vi "Selection ActionBuilder.vi"(9 "Selection Action":T4, 10 "Isolate HPBD":bool, 11 "Chamber Selection":T3) -> (2 "Command Array Out":T1[](array[typedef]), 3 "Action Array Out":T2[](array[typedef]))   [LabVIEW 2011]
uses:
  Selection Action_typdef.ctl
  Chamber Selection_typdef.ctl
  action_typdef.ctl
  command_typdef.ctl
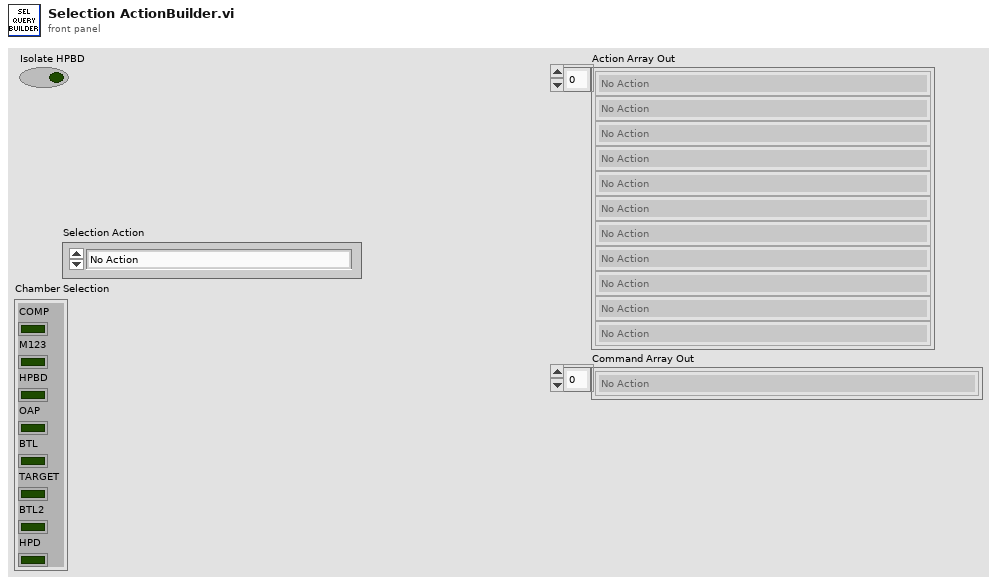
[diagram p1: front panel]
types:
  T1 = typedef "command_typdef.ctl" = enum16{"No Action", "Set GPM Mode LB", "EXIT GPM Mode LB", "Set GPM Mode EC", "EXIT GPM Mode EC", "Set GVM mode LB", "Set GVM Mode EC", "Open LB Backing Valve", "Open EC Backing Valve", "Open EC Roughing Valve", "Open LB Roughing Valve", "Open M123 Roughing Valve", "Close M123 Roughing Valve", "Open Compressor Roughing Valve", "Close Compressor Roughing Valve", "Open BeamDump Roughing Valve", "Close BeamDump Roughing Valve", "Open OAP Roughing Valve", "Close OAP Roughing Valve", "Open BTL Roughing Valve", "Close BTL Roughing Valve", "Open Target Roughing Valve", "Close Target Roughing Valve", "Open BTL2 Roughing Valve", "Close BTL2 Roughing Valve", "Open HPD Roughing Valve", "Close HPD Roughing Valve", "LB Start Roughing Pump ", "EC Start Roughing Pump", "Open COMP Turbo Backing Valve", "Open M123 Turbo Backing Valve", "Open OAP Turbo Backing Valve", "Open HPBD Turbo Backing Valve", "Open BLT Turbo Backing Valve", "Open TARGET1 Turbo Backing Valve", "Open TARGET2 Turbo Backing Valve", "Open BLT2 Turbo Backing Valve", "Open HPD Turbo Backing Valve", "LB Start Turbo Backing Pump", "EC Start Turbo Backing Pump", "Start COMP Turbo Pump", "Start M123 Turbo Pump", "Start OAP Turbo Pump", "Start BTL Turbo Pump", "Start TARGET1 Turbo Pump", "Start TARGET2 Turbo Pump", "Start BTL2 Turbo Pump", "Start HPD Turbo Pump", "Open COMP Turbo Gate Valve", "Open M123 Turbo Gate Valve", "Open OAP Turbo Gate Valve", "Open BTL Turbo Gate Valve", "Open TARGET1 Turbo Gate Valve", "Open TARGET2 Turbo Gate Valve", "Open BTL2 Turbo Gate Valve", "Open HPD Turbo Gate Valve"}
  T2 = typedef "action_typdef.ctl" = enum16{"No Action", "Is EC GPM Mode ON?", "Is EC GPM Mode Off?", "Is EC GVM Mode ON?", "Is EC GVM Off?", "Is  EC GPM or GVM Mode ON?", "Is LB GPM Mode ON?", "Is LB GPM Mode Off?", "Is LB GVM Mode ON?", "Is LB GVM Mode Off?", "Is  LB GPM or GVM Mode ON?", "Is M123 Turbo Gate Valve Opened? ", "Is M123 Turbo Gate Valve Closed?", "Is OAP Turbo Gate Valve Opened?", "Is OAP Turbo Gate Valve Closed?", "Is BTLTurbo Gate Valve Opened?", "Is BTL Turbo Gate Valve Closed?", "Is TARGET Turbo Gate Valve 1Opened?", "Is TARGET1 Turbo Gate Valve Closed?", "Is TARGET Turbo Gate Valve 2 Opened?", "Is TAREGT2 Turbo Gate Valve Closed?", "Is BTL2 Turbo Gate Valve Opened?", "Is BTL2 Turbo Gate Valve Closed?", "Is HPD Turbo Gate Valve Opened?", "Is HPD Turbo Gate Valve Closed?", "Is COMP to M123 gate Valve Opened?", "Is COMP to M123 Valve Closed?", "Is HPBD Gate Valve Opened?", "Is HPBD Gate Valve Closed?", "Is M123 to OAP gate valve opened?", "Is M123 to OAP gate valve closed?", "Is OAP to BLT gate valve opened?", "Is OAP to BTL Gate Valve Closed?", "Is BLT to TARGET gate valve opened?", "Is BTL to TARGET Gate Valve Closed?", "Is TARGET to BLT2 gate valve opened?", "Is TARGET to BTL2 Gate Valve Closed?", "Is BLT2 to HPD gate valve opened?", "Is BTL2 to HPD Gate Valve Closed?", "Is COMP at Atmospheric Pressure?", "Is M123 at Atmospheric Pressure?", "Is BeamDump at Atmospheric Pressure?", "Is OAP at Atmospheric Pressure?", "Is BLT at Atmospheric Pressure", "Is TARGET at Atmospheric Pressure?", "Is BLT2 at Atmospheric Pressure?", "Is HPD at Atmospheric Pressure?", "Is the EC Roughing Pump ON?", "Is the EC Roughing Pump OFF?", "Does the EC Roughing Pump have a fault?", "Is the LB Roughing Pump ON?", "Is the LB Roughing Pump Off?", "Does the LB Roughing Pump have a fault?", "Is the EC Backing Pump ON?", "Is the EC Backing Pump OFF?", "Is the LB Backing Pump ON?", "Is the LB Backing Pump OFF?", "Does the EC Backing Pump have a fault?", "Does the LB Backing Pump have a fault?", "Is the EC Backing Pipe at Atmospheric Pressure", "Is the LB Backing Pipe at Atmospheric Pressure", "Is the EC Backing Manifold at Atmospheric Pressure", "s the LB Backing Manifold at Atmospheric Pressure?", "Is the EC Roughing Pipe at Atmospheric Pressure", "Is the LB Roughing Pipe at Atmospheric Pressure?", "Is the EC Roughing Manifold at Atmospheric Pressure", "Is the LB Roughing Manifold at Atmospheric Pressure", "Is LB Backing Manifold Valve Opened?", "Is EC Backing Manifold Valve Opened?", "Is LB Roughing Manifold Valve Opened?", "Is EC Roughing Manifold Valve Opened?", "Is COMP Roughing Valve Opened?", "Is M123 Roughing Valve Opened?", "Is M123 Roughing Valve Closed?", "Is OAP Roughing Valve Opened?", "Is OAP Roughing Valve Closed?", "Is HPBD Roughing Valve Opened?", "Is HPBD Roughing Valve Closed?", "Is BTL Roughing Valve Opened?", "Is BTL Roughing Valve Closed?", "Is TARGET Roughing Valve Opened?", "Is TARGET Roughing Valve Closed?", "Is BTL2 Roughing Valve Opened?", "Is BTL2 Roughing Valve Closed?", "Is HPD Roughing Valve Opened?", "Is HPD Roughing Valve Closed?", "Is COMP Turbo Backing Valve Opened?", "Is M123 Turbo Backing Valve Opened", "Is HPBD Turbo Backing Valve Opened?", "Is OAP Turbo Backing Valve Opened?", "Is BTL Turbo Backing Valve Opened?", "Is TARGET1 Turbo Backing Valve Opened?", "Is TARGET2 Turbo Backing Valve Opened?", "Is BTL2 Turbo Backing Valve Opened?", "Is HPD Turbo Backing Valve Opened?", "Is M123 Backing at MID-VAC?", "Is OAP Backing at MID-VAC?", "Is TARGET1 Backing at MID-VAC?", "Is TARGET2 Backing at MID-VAC?", "Is BTL Backing at MID-VAC?", "Is BTL2 Backing at MID-VAC?", "Is HPD Backing at MID-VAC?", "Is M123 Turbo in Normal Operation", "Is COMP Turbo in Normal Operation", "Is OAP Turbo in Normal Operation", "Is BTL Turbo in Normal Operation", "Is TARGET1 Turbo in Normal Operation", "Is TARGET2 Turbo in Normal Operation", "Is BTL2 Turbo in Normal Operation", "Is HPD Turbo in Normal Operation", "Is M123 at MID-VAC?", "Is OAP at MID-VAC?", "Is COMP at MID-VAC?", "Is BTL at MID-VAC?", "Is TARGET at MID-VAC?", "Is BTL2 at MID-VAC?", "Is HPD at MID-VAC?"}
  T3 = typedef "Chamber Selection_typdef.ctl" = cluster{"COMP":bool, "M123":bool, "HPBD":bool, "OAP":bool, "BTL":bool, "TARGET":bool, "BTL2":bool, "HPD":bool}
  T4 = typedef "Selection Action_typdef.ctl" = enum16{"No Action", "Check Chamber Pressure", "Check Turbo Gate Valves", "Open Turbo Backing Valves", "Check Turbo Backing Valves", "Check MID-VAC on Chambers", "Start Turbo Pumps", "Check Turbo Normal Operation", "Check Chamber Pressures", "Roughing Valve Selection"}
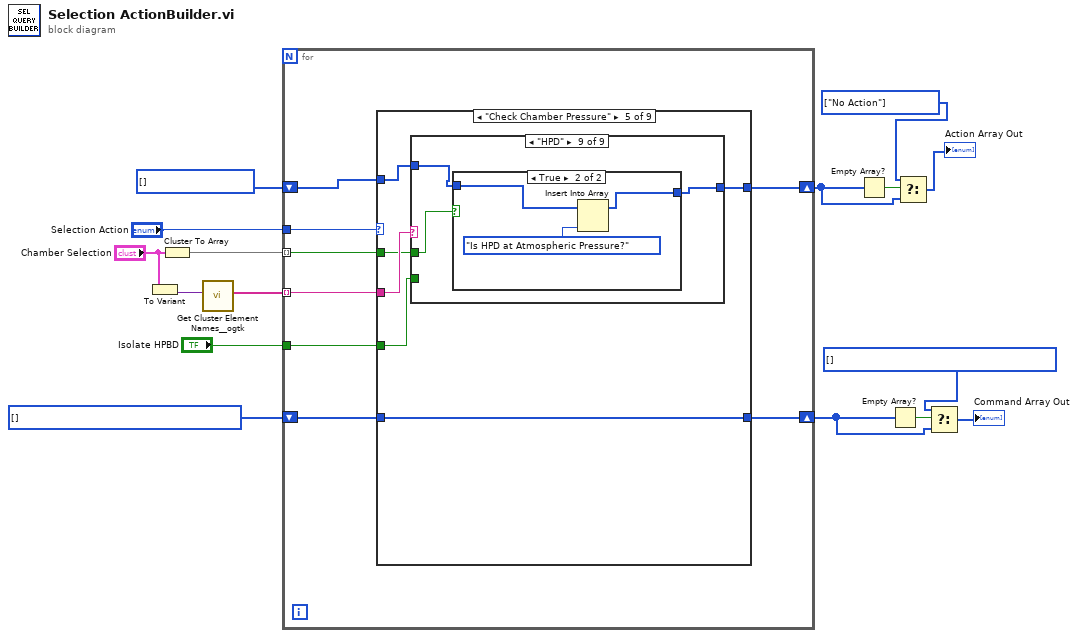
[diagram p0: block diagram]
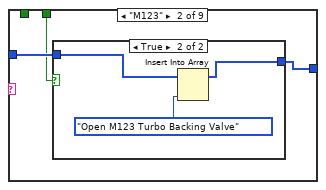
[diagram p4: hidden frame]
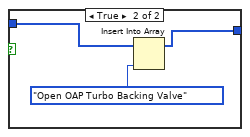
[diagram p7: hidden frame]
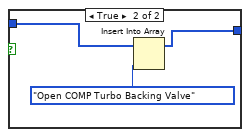
[diagram p9: hidden frame]
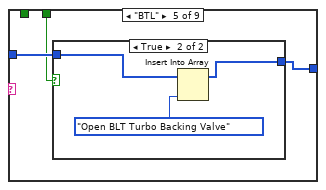
[diagram p10: hidden frame]
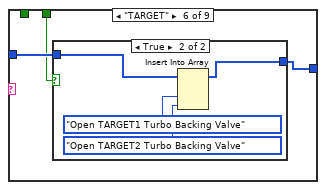
[diagram p12: hidden frame]
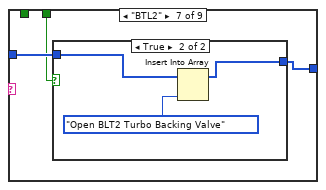
[diagram p14: hidden frame]
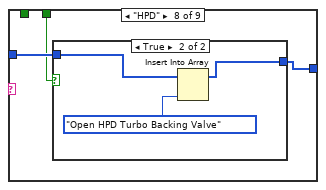
[diagram p16: hidden frame]
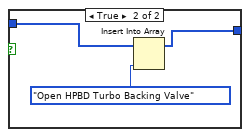
[diagram p20: hidden frame]
diagram:
  w2 = T1[] [] items=["No Action", "Set GPM Mode LB", "EXIT GPM Mode LB", "Set GPM Mode EC", "EXIT GPM Mode EC", "Set GVM mode LB", "Set GVM Mode EC", "Open LB Backing Valve", "Open EC Backing Valve", "Open EC Roughing Valve", "Open LB Roughing Valve", "Open M123 Roughing Valve", "Close M123 Roughing Valve", "Open Compressor Roughing Valve", "Close Compressor Roughing Valve", "Open BeamDump Roughing Valve", "Close BeamDump Roughing Valve", "Open OAP Roughing Valve", "Close OAP Roughing Valve", "Open BTL Roughing Valve", "Close BTL Roughing Valve", "Open Target Roughing Valve", "Close Target Roughing Valve", "Open BTL2 Roughing Valve", "Close BTL2 Roughing Valve", "Open HPD Roughing Valve", "Close HPD Roughing Valve", "LB Start Roughing Pump ", "EC Start Roughing Pump", "Open COMP Turbo Backing Valve", "Open M123 Turbo Backing Valve", "Open OAP Turbo Backing Valve", "Open HPBD Turbo Backing Valve", "Open BLT Turbo Backing Valve", "Open TARGET1 Turbo Backing Valve", "Open TARGET2 Turbo Backing Valve", "Open BLT2 Turbo Backing Valve", "Open HPD Turbo Backing Valve", "LB Start Turbo Backing Pump", "EC Start Turbo Backing Pump", "Start COMP Turbo Pump", "Start M123 Turbo Pump", "Start OAP Turbo Pump", "Start BTL Turbo Pump", "Start TARGET1 Turbo Pump", "Start TARGET2 Turbo Pump", "Start BTL2 Turbo Pump", "Start HPD Turbo Pump", "Open COMP Turbo Gate Valve", "Open M123 Turbo Gate Valve", "Open OAP Turbo Gate Valve", "Open BTL Turbo Gate Valve", "Open TARGET1 Turbo Gate Valve", "Open TARGET2 Turbo Gate Valve", "Open BTL2 Turbo Gate Valve", "Open HPD Turbo Gate Valve"]
  w5 = T1[] [] items=["No Action", "Set GPM Mode LB", "EXIT GPM Mode LB", "Set GPM Mode EC", "EXIT GPM Mode EC", "Set GVM mode LB", "Set GVM Mode EC", "Open LB Backing Valve", "Open EC Backing Valve", "Open EC Roughing Valve", "Open LB Roughing Valve", "Open M123 Roughing Valve", "Close M123 Roughing Valve", "Open Compressor Roughing Valve", "Close Compressor Roughing Valve", "Open BeamDump Roughing Valve", "Close BeamDump Roughing Valve", "Open OAP Roughing Valve", "Close OAP Roughing Valve", "Open BTL Roughing Valve", "Close BTL Roughing Valve", "Open Target Roughing Valve", "Close Target Roughing Valve", "Open BTL2 Roughing Valve", "Close BTL2 Roughing Valve", "Open HPD Roughing Valve", "Close HPD Roughing Valve", "LB Start Roughing Pump ", "EC Start Roughing Pump", "Open COMP Turbo Backing Valve", "Open M123 Turbo Backing Valve", "Open OAP Turbo Backing Valve", "Open HPBD Turbo Backing Valve", "Open BLT Turbo Backing Valve", "Open TARGET1 Turbo Backing Valve", "Open TARGET2 Turbo Backing Valve", "Open BLT2 Turbo Backing Valve", "Open HPD Turbo Backing Valve", "LB Start Turbo Backing Pump", "EC Start Turbo Backing Pump", "Start COMP Turbo Pump", "Start M123 Turbo Pump", "Start OAP Turbo Pump", "Start BTL Turbo Pump", "Start TARGET1 Turbo Pump", "Start TARGET2 Turbo Pump", "Start BTL2 Turbo Pump", "Start HPD Turbo Pump", "Open COMP Turbo Gate Valve", "Open M123 Turbo Gate Valve", "Open OAP Turbo Gate Valve", "Open BTL Turbo Gate Valve", "Open TARGET1 Turbo Gate Valve", "Open TARGET2 Turbo Gate Valve", "Open BTL2 Turbo Gate Valve", "Open HPD Turbo Gate Valve"]
  w7 = T2[] [enum."No Action"] items=["No Action", "Is EC GPM Mode ON?", "Is EC GPM Mode Off?", "Is EC GVM Mode ON?", "Is EC GVM Off?", "Is  EC GPM or GVM Mode ON?", "Is LB GPM Mode ON?", "Is LB GPM Mode Off?", "Is LB GVM Mode ON?", "Is LB GVM Mode Off?", "Is  LB GPM or GVM Mode ON?", "Is M123 Turbo Gate Valve Opened? ", "Is M123 Turbo Gate Valve Closed?", "Is OAP Turbo Gate Valve Opened?", "Is OAP Turbo Gate Valve Closed?", "Is BTLTurbo Gate Valve Opened?", "Is BTL Turbo Gate Valve Closed?", "Is TARGET Turbo Gate Valve 1Opened?", "Is TARGET1 Turbo Gate Valve Closed?", "Is TARGET Turbo Gate Valve 2 Opened?", "Is TAREGT2 Turbo Gate Valve Closed?", "Is BTL2 Turbo Gate Valve Opened?", "Is BTL2 Turbo Gate Valve Closed?", "Is HPD Turbo Gate Valve Opened?", "Is HPD Turbo Gate Valve Closed?", "Is COMP to M123 gate Valve Opened?", "Is COMP to M123 Valve Closed?", "Is HPBD Gate Valve Opened?", "Is HPBD Gate Valve Closed?", "Is M123 to OAP gate valve opened?", "Is M123 to OAP gate valve closed?", "Is OAP to BLT gate valve opened?", "Is OAP to BTL Gate Valve Closed?", "Is BLT to TARGET gate valve opened?", "Is BTL to TARGET Gate Valve Closed?", "Is TARGET to BLT2 gate valve opened?", "Is TARGET to BTL2 Gate Valve Closed?", "Is BLT2 to HPD gate valve opened?", "Is BTL2 to HPD Gate Valve Closed?", "Is COMP at Atmospheric Pressure?", "Is M123 at Atmospheric Pressure?", "Is BeamDump at Atmospheric Pressure?", "Is OAP at Atmospheric Pressure?", "Is BLT at Atmospheric Pressure", "Is TARGET at Atmospheric Pressure?", "Is BLT2 at Atmospheric Pressure?", "Is HPD at Atmospheric Pressure?", "Is the EC Roughing Pump ON?", "Is the EC Roughing Pump OFF?", "Does the EC Roughing Pump have a fault?", "Is the LB Roughing Pump ON?", "Is the LB Roughing Pump Off?", "Does the LB Roughing Pump have a fault?", "Is the EC Backing Pump ON?", "Is the EC Backing Pump OFF?", "Is the LB Backing Pump ON?", "Is the LB Backing Pump OFF?", "Does the EC Backing Pump have a fault?", "Does the LB Backing Pump have a fault?", "Is the EC Backing Pipe at Atmospheric Pressure", "Is the LB Backing Pipe at Atmospheric Pressure", "Is the EC Backing Manifold at Atmospheric Pressure", "s the LB Backing Manifold at Atmospheric Pressure?", "Is the EC Roughing Pipe at Atmospheric Pressure", "Is the LB Roughing Pipe at Atmospheric Pressure?", "Is the EC Roughing Manifold at Atmospheric Pressure", "Is the LB Roughing Manifold at Atmospheric Pressure", "Is LB Backing Manifold Valve Opened?", "Is EC Backing Manifold Valve Opened?", "Is LB Roughing Manifold Valve Opened?", "Is EC Roughing Manifold Valve Opened?", "Is COMP Roughing Valve Opened?", "Is M123 Roughing Valve Opened?", "Is M123 Roughing Valve Closed?", "Is OAP Roughing Valve Opened?", "Is OAP Roughing Valve Closed?", "Is HPBD Roughing Valve Opened?", "Is HPBD Roughing Valve Closed?", "Is BTL Roughing Valve Opened?", "Is BTL Roughing Valve Closed?", "Is TARGET Roughing Valve Opened?", "Is TARGET Roughing Valve Closed?", "Is BTL2 Roughing Valve Opened?", "Is BTL2 Roughing Valve Closed?", "Is HPD Roughing Valve Opened?", "Is HPD Roughing Valve Closed?", "Is COMP Turbo Backing Valve Opened?", "Is M123 Turbo Backing Valve Opened", "Is HPBD Turbo Backing Valve Opened?", "Is OAP Turbo Backing Valve Opened?", "Is BTL Turbo Backing Valve Opened?", "Is TARGET1 Turbo Backing Valve Opened?", "Is TARGET2 Turbo Backing Valve Opened?", "Is BTL2 Turbo Backing Valve Opened?", "Is HPD Turbo Backing Valve Opened?", "Is M123 Backing at MID-VAC?", "Is OAP Backing at MID-VAC?", "Is TARGET1 Backing at MID-VAC?", "Is TARGET2 Backing at MID-VAC?", "Is BTL Backing at MID-VAC?", "Is BTL2 Backing at MID-VAC?", "Is HPD Backing at MID-VAC?", "Is M123 Turbo in Normal Operation", "Is COMP Turbo in Normal Operation", "Is OAP Turbo in Normal Operation", "Is BTL Turbo in Normal Operation", "Is TARGET1 Turbo in Normal Operation", "Is TARGET2 Turbo in Normal Operation", "Is BTL2 Turbo in Normal Operation", "Is HPD Turbo in Normal Operation", "Is M123 at MID-VAC?", "Is OAP at MID-VAC?", "Is COMP at MID-VAC?", "Is BTL at MID-VAC?", "Is TARGET at MID-VAC?", "Is BTL2 at MID-VAC?", "Is HPD at MID-VAC?"]
  w10 = T2[] [] items=["No Action", "Is EC GPM Mode ON?", "Is EC GPM Mode Off?", "Is EC GVM Mode ON?", "Is EC GVM Off?", "Is  EC GPM or GVM Mode ON?", "Is LB GPM Mode ON?", "Is LB GPM Mode Off?", "Is LB GVM Mode ON?", "Is LB GVM Mode Off?", "Is  LB GPM or GVM Mode ON?", "Is M123 Turbo Gate Valve Opened? ", "Is M123 Turbo Gate Valve Closed?", "Is OAP Turbo Gate Valve Opened?", "Is OAP Turbo Gate Valve Closed?", "Is BTLTurbo Gate Valve Opened?", "Is BTL Turbo Gate Valve Closed?", "Is TARGET Turbo Gate Valve 1Opened?", "Is TARGET1 Turbo Gate Valve Closed?", "Is TARGET Turbo Gate Valve 2 Opened?", "Is TAREGT2 Turbo Gate Valve Closed?", "Is BTL2 Turbo Gate Valve Opened?", "Is BTL2 Turbo Gate Valve Closed?", "Is HPD Turbo Gate Valve Opened?", "Is HPD Turbo Gate Valve Closed?", "Is COMP to M123 gate Valve Opened?", "Is COMP to M123 Valve Closed?", "Is HPBD Gate Valve Opened?", "Is HPBD Gate Valve Closed?", "Is M123 to OAP gate valve opened?", "Is M123 to OAP gate valve closed?", "Is OAP to BLT gate valve opened?", "Is OAP to BTL Gate Valve Closed?", "Is BLT to TARGET gate valve opened?", "Is BTL to TARGET Gate Valve Closed?", "Is TARGET to BLT2 gate valve opened?", "Is TARGET to BTL2 Gate Valve Closed?", "Is BLT2 to HPD gate valve opened?", "Is BTL2 to HPD Gate Valve Closed?", "Is COMP at Atmospheric Pressure?", "Is M123 at Atmospheric Pressure?", "Is BeamDump at Atmospheric Pressure?", "Is OAP at Atmospheric Pressure?", "Is BLT at Atmospheric Pressure", "Is TARGET at Atmospheric Pressure?", "Is BLT2 at Atmospheric Pressure?", "Is HPD at Atmospheric Pressure?", "Is the EC Roughing Pump ON?", "Is the EC Roughing Pump OFF?", "Does the EC Roughing Pump have a fault?", "Is the LB Roughing Pump ON?", "Is the LB Roughing Pump Off?", "Does the LB Roughing Pump have a fault?", "Is the EC Backing Pump ON?", "Is the EC Backing Pump OFF?", "Is the LB Backing Pump ON?", "Is the LB Backing Pump OFF?", "Does the EC Backing Pump have a fault?", "Does the LB Backing Pump have a fault?", "Is the EC Backing Pipe at Atmospheric Pressure", "Is the LB Backing Pipe at Atmospheric Pressure", "Is the EC Backing Manifold at Atmospheric Pressure", "s the LB Backing Manifold at Atmospheric Pressure?", "Is the EC Roughing Pipe at Atmospheric Pressure", "Is the LB Roughing Pipe at Atmospheric Pressure?", "Is the EC Roughing Manifold at Atmospheric Pressure", "Is the LB Roughing Manifold at Atmospheric Pressure", "Is LB Backing Manifold Valve Opened?", "Is EC Backing Manifold Valve Opened?", "Is LB Roughing Manifold Valve Opened?", "Is EC Roughing Manifold Valve Opened?", "Is COMP Roughing Valve Opened?", "Is M123 Roughing Valve Opened?", "Is M123 Roughing Valve Closed?", "Is OAP Roughing Valve Opened?", "Is OAP Roughing Valve Closed?", "Is HPBD Roughing Valve Opened?", "Is HPBD Roughing Valve Closed?", "Is BTL Roughing Valve Opened?", "Is BTL Roughing Valve Closed?", "Is TARGET Roughing Valve Opened?", "Is TARGET Roughing Valve Closed?", "Is BTL2 Roughing Valve Opened?", "Is BTL2 Roughing Valve Closed?", "Is HPD Roughing Valve Opened?", "Is HPD Roughing Valve Closed?", "Is COMP Turbo Backing Valve Opened?", "Is M123 Turbo Backing Valve Opened", "Is HPBD Turbo Backing Valve Opened?", "Is OAP Turbo Backing Valve Opened?", "Is BTL Turbo Backing Valve Opened?", "Is TARGET1 Turbo Backing Valve Opened?", "Is TARGET2 Turbo Backing Valve Opened?", "Is BTL2 Turbo Backing Valve Opened?", "Is HPD Turbo Backing Valve Opened?", "Is M123 Backing at MID-VAC?", "Is OAP Backing at MID-VAC?", "Is TARGET1 Backing at MID-VAC?", "Is TARGET2 Backing at MID-VAC?", "Is BTL Backing at MID-VAC?", "Is BTL2 Backing at MID-VAC?", "Is HPD Backing at MID-VAC?", "Is M123 Turbo in Normal Operation", "Is COMP Turbo in Normal Operation", "Is OAP Turbo in Normal Operation", "Is BTL Turbo in Normal Operation", "Is TARGET1 Turbo in Normal Operation", "Is TARGET2 Turbo in Normal Operation", "Is BTL2 Turbo in Normal Operation", "Is HPD Turbo in Normal Operation", "Is M123 at MID-VAC?", "Is OAP at MID-VAC?", "Is COMP at MID-VAC?", "Is BTL at MID-VAC?", "Is TARGET at MID-VAC?", "Is BTL2 at MID-VAC?", "Is HPD at MID-VAC?"]
  n1 = To Variant(anything="Chamber Selection") -> (Variant=w13:variant)
  n2 = Cluster To Array(cluster="Chamber Selection") -> (array=w16:bool[])
  n3 = call <userlib>:"Get Cluster Element Names__ogtk.vi"("Cluster"=w13) -> ("Element Names"=w12:string[])  [unwired: 9 in, 1 out]
  n4 = for {
    tunnel: w16 -> [w23] mode=indexing
    tunnel: "Selection Action" -> [w24]
    tunnel: w12 -> [w22] mode=indexing
    tunnel: "Isolate HPBD" -> [w21]
    shift-right: [w19] -> w6
    shift-left: w10 -> [w20]
    shift-right: [w17] -> w3
    shift-left: w5 -> [w18]
    n5 = case shown="\"Check Chamber Pressure\"" w24 {
      tunnel: w23 -> [_ w29 w98 _ w170 w238 w304 w371 w440]
      tunnel: w22 -> [_ w32 w101 _ w172 w240 w306 w373 w442]
      tunnel: w21 -> [_ w28 w97 _ w171 w239 w305 w372 w441]
      tunnel: w20 -> [w26 w27 w96 _ w169 w237 w303 w370 w439]
      tunnel: [w26 w27 w96 w166 w168 w236 w302 w369 w438] -> w19
      tunnel: w18 -> [w25 w31 w100 w165 w167 w235 w301 w368 w437]
      tunnel: [w25 w30 w99 w165 w167 w235 w301 w368 w437] -> w17
      frame "Check Turbo Gate Valves" {
      }
      frame "Open Turbo Backing Valves" {
        n6 = case shown="\"False\", Default" w32 {
          tunnel: w31 -> [w33 w36 w43 w50 w57 w64 w72 w79 w87]
          tunnel: [w33 w35 w42 w49 w56 w63 w71 w78 w86] -> w30
          tunnel: w29 -> [_ w34 w41 w48 w55 w62 w70 w77 w84]
          tunnel: w28 -> [_ _ _ _ _ _ _ _ w85]
          frame "False", Default {
          }
          frame "M123" {
            n7 = case shown="True" w34 {
              tunnel: w36 -> [w37 w40]
              tunnel: [w37 w39] -> w35
              frame False {
              }
              frame True {
                n8 = Insert Into Array(array=w40, new element=command_typdef."Open M123 Turbo Backing Valve" ("Command")) -> (w39:T1[])  [unwired: 1 in]
              }
            }
          }
          frame "OAP" {
            n9 = case shown="False" w41 {
              tunnel: w43 -> [w44 w47]
              tunnel: [w44 w46] -> w42
              frame False {
              }
              frame True {
                n10 = Insert Into Array(array=w47, new element=command_typdef."Open OAP Turbo Backing Valve" ("Command")) -> (w46:T1[])  [unwired: 1 in]
              }
            }
          }
          frame "COMP" {
            n11 = case shown="False" w48 {
              tunnel: w50 -> [w51 w54]
              tunnel: [w51 w53] -> w49
              frame False {
              }
              frame True {
                n12 = Insert Into Array(array=w54, new element=command_typdef."Open COMP Turbo Backing Valve" ("Command")) -> (w53:T1[])  [unwired: 1 in]
              }
            }
          }
          frame "BTL" {
            n13 = case shown="True" w55 {
              tunnel: w57 -> [w58 w61]
              tunnel: [w58 w60] -> w56
              frame False {
              }
              frame True {
                n14 = Insert Into Array(array=w61, new element=command_typdef."Open BLT Turbo Backing Valve" ("Command")) -> (w60:T1[])  [unwired: 1 in]
              }
            }
          }
          frame "TARGET" {
            n15 = case shown="True" w62 {
              tunnel: w64 -> [w65 w69]
              tunnel: [w65 w68] -> w63
              frame False {
              }
              frame True {
                n16 = Insert Into Array(array=w69, new element #1=command_typdef."Open TARGET1 Turbo Backing Valve" ("Command"), new element #2=command_typdef."Open TARGET2 Turbo Backing Valve" ("Command")) -> (w68:T1[])  [unwired: 1 in]
              }
            }
          }
          frame "BTL2" {
            n17 = case shown="True" w70 {
              tunnel: w72 -> [w73 w76]
              tunnel: [w73 w75] -> w71
              frame False {
              }
              frame True {
                n18 = Insert Into Array(array=w76, new element=command_typdef."Open BLT2 Turbo Backing Valve" ("Command")) -> (w75:T1[])  [unwired: 1 in]
              }
            }
          }
          frame "HPD" {
            n19 = case shown="True" w77 {
              tunnel: w79 -> [w80 w83]
              tunnel: [w80 w82] -> w78
              frame False {
              }
              frame True {
                n20 = Insert Into Array(array=w83, new element=command_typdef."Open HPD Turbo Backing Valve" ("Command")) -> (w82:T1[])  [unwired: 1 in]
              }
            }
          }
          frame "HPBD" {
            n21 = case shown="True" w85 {
              tunnel: w87 -> [w90 w95]
              tunnel: [w89 w95] -> w86
              tunnel: w84 -> [w88 _]
              frame False {
                n22 = case shown="False" w88 {
                  tunnel: w90 -> [w91 w94]
                  tunnel: [w91 w93] -> w89
                  frame False {
                  }
                  frame True {
                    n23 = Insert Into Array(array=w94, new element=command_typdef."Open HPBD Turbo Backing Valve" ("Command")) -> (w93:T1[])  [unwired: 1 in]
                  }
                }
              }
              frame True {
              }
            }
          }
        }
      }
      frame "Start Turbo Pumps" {
        n24 = case shown="\"M123\"" w101 {
          tunnel: w100 -> [w102 w105 w112 w119 w126 w133 w141 w148 w156]
          tunnel: [w102 w104 w111 w118 w125 w132 w140 w147 w155] -> w99
          tunnel: w98 -> [_ w103 w110 w117 w124 w131 w139 w146 w153]
          tunnel: w97 -> [_ _ _ _ _ _ _ _ w154]
          frame "False", Default {
          }
          frame "M123" {
            n25 = case shown="True" w103 {
              tunnel: w105 -> [w106 w109]
              tunnel: [w106 w108] -> w104
              frame False {
              }
              frame True {
                n26 = Insert Into Array(array=w109, new element=command_typdef."Start M123 Turbo Pump" ("Command")) -> (w108:T1[])  [unwired: 1 in]
              }
            }
          }
          frame "OAP" {
            n27 = case shown="True" w110 {
              tunnel: w112 -> [w113 w116]
              tunnel: [w113 w115] -> w111
              frame False {
              }
              frame True {
                n28 = Insert Into Array(array=w116, new element=command_typdef."Start OAP Turbo Pump" ("Command")) -> (w115:T1[])  [unwired: 1 in]
              }
            }
          }
          frame "COMP" {
            n29 = case shown="True" w117 {
              tunnel: w119 -> [w120 w123]
              tunnel: [w120 w122] -> w118
              frame False {
              }
              frame True {
                n30 = Insert Into Array(array=w123, new element=command_typdef."Start COMP Turbo Pump" ("Command")) -> (w122:T1[])  [unwired: 1 in]
              }
            }
          }
          frame "BTL" {
            n31 = case shown="True" w124 {
              tunnel: w126 -> [w127 w130]
              tunnel: [w127 w129] -> w125
              frame False {
              }
              frame True {
                n32 = Insert Into Array(array=w130, new element=command_typdef."Start BTL Turbo Pump" ("Command")) -> (w129:T1[])  [unwired: 1 in]
              }
            }
          }
          frame "TARGET" {
            n33 = case shown="True" w131 {
              tunnel: w133 -> [w134 w138]
              tunnel: [w134 w137] -> w132
              frame False {
              }
              frame True {
                n34 = Insert Into Array(array=w138, new element #1=command_typdef."Start TARGET1 Turbo Pump" ("Command"), new element #2=command_typdef."Start TARGET2 Turbo Pump" ("Command")) -> (w137:T1[])  [unwired: 1 in]
              }
            }
          }
          frame "BTL2" {
            n35 = case shown="True" w139 {
              tunnel: w141 -> [w142 w145]
              tunnel: [w142 w144] -> w140
              frame False {
              }
              frame True {
                n36 = Insert Into Array(array=w145, new element=command_typdef."Start BTL2 Turbo Pump" ("Command")) -> (w144:T1[])  [unwired: 1 in]
              }
            }
          }
          frame "HPD" {
            n37 = case shown="True" w146 {
              tunnel: w148 -> [w149 w152]
              tunnel: [w149 w151] -> w147
              frame False {
              }
              frame True {
                n38 = Insert Into Array(array=w152, new element=command_typdef."Start HPD Turbo Pump" ("Command")) -> (w151:T1[])  [unwired: 1 in]
              }
            }
          }
          frame "HPBD" {
            n39 = case shown="True" w154 {
              tunnel: w156 -> [w159 w164]
              tunnel: [w158 w164] -> w155
              tunnel: w153 -> [w157 _]
              frame False {
                n40 = case shown="False" w157 {
                  tunnel: w159 -> [w160 w163]
                  tunnel: [w160 w162] -> w158
                  frame False {
                  }
                  frame True {
                    n41 = Insert Into Array(array=w163, new element=command_typdef."Open HPBD Turbo Backing Valve" ("Command")) -> (w162:T1[])  [unwired: 1 in]
                  }
                }
              }
              frame True {
              }
            }
          }
        }
      }
      frame "No Action", Default {
        w166 = T2[] [enum."No Action"] items=["No Action", "Is EC GPM Mode ON?", "Is EC GPM Mode Off?", "Is EC GVM Mode ON?", "Is EC GVM Off?", "Is  EC GPM or GVM Mode ON?", "Is LB GPM Mode ON?", "Is LB GPM Mode Off?", "Is LB GVM Mode ON?", "Is LB GVM Mode Off?", "Is  LB GPM or GVM Mode ON?", "Is M123 Turbo Gate Valve Opened? ", "Is M123 Turbo Gate Valve Closed?", "Is OAP Turbo Gate Valve Opened?", "Is OAP Turbo Gate Valve Closed?", "Is BTLTurbo Gate Valve Opened?", "Is BTL Turbo Gate Valve Closed?", "Is TARGET Turbo Gate Valve 1Opened?", "Is TARGET1 Turbo Gate Valve Closed?", "Is TARGET Turbo Gate Valve 2 Opened?", "Is TAREGT2 Turbo Gate Valve Closed?", "Is BTL2 Turbo Gate Valve Opened?", "Is BTL2 Turbo Gate Valve Closed?", "Is HPD Turbo Gate Valve Opened?", "Is HPD Turbo Gate Valve Closed?", "Is COMP to M123 gate Valve Opened?", "Is COMP to M123 Valve Closed?", "Is HPBD Gate Valve Opened?", "Is HPBD Gate Valve Closed?", "Is M123 to OAP gate valve opened?", "Is M123 to OAP gate valve closed?", "Is OAP to BLT gate valve opened?", "Is OAP to BTL Gate Valve Closed?", "Is BLT to TARGET gate valve opened?", "Is BTL to TARGET Gate Valve Closed?", "Is TARGET to BLT2 gate valve opened?", "Is TARGET to BTL2 Gate Valve Closed?", "Is BLT2 to HPD gate valve opened?", "Is BTL2 to HPD Gate Valve Closed?", "Is COMP at Atmospheric Pressure?", "Is M123 at Atmospheric Pressure?", "Is BeamDump at Atmospheric Pressure?", "Is OAP at Atmospheric Pressure?", "Is BLT at Atmospheric Pressure", "Is TARGET at Atmospheric Pressure?", "Is BLT2 at Atmospheric Pressure?", "Is HPD at Atmospheric Pressure?", "Is the EC Roughing Pump ON?", "Is the EC Roughing Pump OFF?", "Does the EC Roughing Pump have a fault?", "Is the LB Roughing Pump ON?", "Is the LB Roughing Pump Off?", "Does the LB Roughing Pump have a fault?", "Is the EC Backing Pump ON?", "Is the EC Backing Pump OFF?", "Is the LB Backing Pump ON?", "Is the LB Backing Pump OFF?", "Does the EC Backing Pump have a fault?", "Does the LB Backing Pump have a fault?", "Is the EC Backing Pipe at Atmospheric Pressure", "Is the LB Backing Pipe at Atmospheric Pressure", "Is the EC Backing Manifold at Atmospheric Pressure", "s the LB Backing Manifold at Atmospheric Pressure?", "Is the EC Roughing Pipe at Atmospheric Pressure", "Is the LB Roughing Pipe at Atmospheric Pressure?", "Is the EC Roughing Manifold at Atmospheric Pressure", "Is the LB Roughing Manifold at Atmospheric Pressure", "Is LB Backing Manifold Valve Opened?", "Is EC Backing Manifold Valve Opened?", "Is LB Roughing Manifold Valve Opened?", "Is EC Roughing Manifold Valve Opened?", "Is COMP Roughing Valve Opened?", "Is M123 Roughing Valve Opened?", "Is M123 Roughing Valve Closed?", "Is OAP Roughing Valve Opened?", "Is OAP Roughing Valve Closed?", "Is HPBD Roughing Valve Opened?", "Is HPBD Roughing Valve Closed?", "Is BTL Roughing Valve Opened?", "Is BTL Roughing Valve Closed?", "Is TARGET Roughing Valve Opened?", "Is TARGET Roughing Valve Closed?", "Is BTL2 Roughing Valve Opened?", "Is BTL2 Roughing Valve Closed?", "Is HPD Roughing Valve Opened?", "Is HPD Roughing Valve Closed?", "Is COMP Turbo Backing Valve Opened?", "Is M123 Turbo Backing Valve Opened", "Is HPBD Turbo Backing Valve Opened?", "Is OAP Turbo Backing Valve Opened?", "Is BTL Turbo Backing Valve Opened?", "Is TARGET1 Turbo Backing Valve Opened?", "Is TARGET2 Turbo Backing Valve Opened?", "Is BTL2 Turbo Backing Valve Opened?", "Is HPD Turbo Backing Valve Opened?", "Is M123 Backing at MID-VAC?", "Is OAP Backing at MID-VAC?", "Is TARGET1 Backing at MID-VAC?", "Is TARGET2 Backing at MID-VAC?", "Is BTL Backing at MID-VAC?", "Is BTL2 Backing at MID-VAC?", "Is HPD Backing at MID-VAC?", "Is M123 Turbo in Normal Operation", "Is COMP Turbo in Normal Operation", "Is OAP Turbo in Normal Operation", "Is BTL Turbo in Normal Operation", "Is TARGET1 Turbo in Normal Operation", "Is TARGET2 Turbo in Normal Operation", "Is BTL2 Turbo in Normal Operation", "Is HPD Turbo in Normal Operation", "Is M123 at MID-VAC?", "Is OAP at MID-VAC?", "Is COMP at MID-VAC?", "Is BTL at MID-VAC?", "Is TARGET at MID-VAC?", "Is BTL2 at MID-VAC?", "Is HPD at MID-VAC?"]
      }
      frame "Check Chamber Pressure" {
        n42 = case shown="\"HPD\"" w172 {
          tunnel: w171 -> [_ _ _ w188 _ _ _ _ _]
          tunnel: w170 -> [_ w175 w183 w190 w200 w207 w214 w221 w230]
          tunnel: w169 -> [_ w176 w182 w189 w202 w209 w216 w223 w229]
          tunnel: [w173 w174 w181 w191 w201 w208 w215 w222 w228] -> w168
          frame "False", Default {
            w173 = T2[] [enum."No Action"] items=["No Action", "Is EC GPM Mode ON?", "Is EC GPM Mode Off?", "Is EC GVM Mode ON?", "Is EC GVM Off?", "Is  EC GPM or GVM Mode ON?", "Is LB GPM Mode ON?", "Is LB GPM Mode Off?", "Is LB GVM Mode ON?", "Is LB GVM Mode Off?", "Is  LB GPM or GVM Mode ON?", "Is M123 Turbo Gate Valve Opened? ", "Is M123 Turbo Gate Valve Closed?", "Is OAP Turbo Gate Valve Opened?", "Is OAP Turbo Gate Valve Closed?", "Is BTLTurbo Gate Valve Opened?", "Is BTL Turbo Gate Valve Closed?", "Is TARGET Turbo Gate Valve 1Opened?", "Is TARGET1 Turbo Gate Valve Closed?", "Is TARGET Turbo Gate Valve 2 Opened?", "Is TAREGT2 Turbo Gate Valve Closed?", "Is BTL2 Turbo Gate Valve Opened?", "Is BTL2 Turbo Gate Valve Closed?", "Is HPD Turbo Gate Valve Opened?", "Is HPD Turbo Gate Valve Closed?", "Is COMP to M123 gate Valve Opened?", "Is COMP to M123 Valve Closed?", "Is HPBD Gate Valve Opened?", "Is HPBD Gate Valve Closed?", "Is M123 to OAP gate valve opened?", "Is M123 to OAP gate valve closed?", "Is OAP to BLT gate valve opened?", "Is OAP to BTL Gate Valve Closed?", "Is BLT to TARGET gate valve opened?", "Is BTL to TARGET Gate Valve Closed?", "Is TARGET to BLT2 gate valve opened?", "Is TARGET to BTL2 Gate Valve Closed?", "Is BLT2 to HPD gate valve opened?", "Is BTL2 to HPD Gate Valve Closed?", "Is COMP at Atmospheric Pressure?", "Is M123 at Atmospheric Pressure?", "Is BeamDump at Atmospheric Pressure?", "Is OAP at Atmospheric Pressure?", "Is BLT at Atmospheric Pressure", "Is TARGET at Atmospheric Pressure?", "Is BLT2 at Atmospheric Pressure?", "Is HPD at Atmospheric Pressure?", "Is the EC Roughing Pump ON?", "Is the EC Roughing Pump OFF?", "Does the EC Roughing Pump have a fault?", "Is the LB Roughing Pump ON?", "Is the LB Roughing Pump Off?", "Does the LB Roughing Pump have a fault?", "Is the EC Backing Pump ON?", "Is the EC Backing Pump OFF?", "Is the LB Backing Pump ON?", "Is the LB Backing Pump OFF?", "Does the EC Backing Pump have a fault?", "Does the LB Backing Pump have a fault?", "Is the EC Backing Pipe at Atmospheric Pressure", "Is the LB Backing Pipe at Atmospheric Pressure", "Is the EC Backing Manifold at Atmospheric Pressure", "s the LB Backing Manifold at Atmospheric Pressure?", "Is the EC Roughing Pipe at Atmospheric Pressure", "Is the LB Roughing Pipe at Atmospheric Pressure?", "Is the EC Roughing Manifold at Atmospheric Pressure", "Is the LB Roughing Manifold at Atmospheric Pressure", "Is LB Backing Manifold Valve Opened?", "Is EC Backing Manifold Valve Opened?", "Is LB Roughing Manifold Valve Opened?", "Is EC Roughing Manifold Valve Opened?", "Is COMP Roughing Valve Opened?", "Is M123 Roughing Valve Opened?", "Is M123 Roughing Valve Closed?", "Is OAP Roughing Valve Opened?", "Is OAP Roughing Valve Closed?", "Is HPBD Roughing Valve Opened?", "Is HPBD Roughing Valve Closed?", "Is BTL Roughing Valve Opened?", "Is BTL Roughing Valve Closed?", "Is TARGET Roughing Valve Opened?", "Is TARGET Roughing Valve Closed?", "Is BTL2 Roughing Valve Opened?", "Is BTL2 Roughing Valve Closed?", "Is HPD Roughing Valve Opened?", "Is HPD Roughing Valve Closed?", "Is COMP Turbo Backing Valve Opened?", "Is M123 Turbo Backing Valve Opened", "Is HPBD Turbo Backing Valve Opened?", "Is OAP Turbo Backing Valve Opened?", "Is BTL Turbo Backing Valve Opened?", "Is TARGET1 Turbo Backing Valve Opened?", "Is TARGET2 Turbo Backing Valve Opened?", "Is BTL2 Turbo Backing Valve Opened?", "Is HPD Turbo Backing Valve Opened?", "Is M123 Backing at MID-VAC?", "Is OAP Backing at MID-VAC?", "Is TARGET1 Backing at MID-VAC?", "Is TARGET2 Backing at MID-VAC?", "Is BTL Backing at MID-VAC?", "Is BTL2 Backing at MID-VAC?", "Is HPD Backing at MID-VAC?", "Is M123 Turbo in Normal Operation", "Is COMP Turbo in Normal Operation", "Is OAP Turbo in Normal Operation", "Is BTL Turbo in Normal Operation", "Is TARGET1 Turbo in Normal Operation", "Is TARGET2 Turbo in Normal Operation", "Is BTL2 Turbo in Normal Operation", "Is HPD Turbo in Normal Operation", "Is M123 at MID-VAC?", "Is OAP at MID-VAC?", "Is COMP at MID-VAC?", "Is BTL at MID-VAC?", "Is TARGET at MID-VAC?", "Is BTL2 at MID-VAC?", "Is HPD at MID-VAC?"]
          }
          frame "COMP" {
            n43 = case shown="True" w175 {
              tunnel: w176 -> [w177 w180]
              tunnel: [w177 w178] -> w174
              frame False {
              }
              frame True {
                n44 = Insert Into Array(array=w180, new element=action_typdef."Is COMP at Atmospheric Pressure?" ("action")) -> (w178:T2[])  [unwired: 1 in]
              }
            }
          }
          frame "M123" {
            n45 = case shown="True" w183 {
              tunnel: w182 -> [w184 w186]
              tunnel: [w184 w185] -> w181
              frame False {
              }
              frame True {
                n46 = Insert Into Array(array=w186, new element=action_typdef."Is M123 at Atmospheric Pressure?" ("action")) -> (w185:T2[])  [unwired: 1 in]
              }
            }
          }
          frame "HPBD" {
            n47 = case shown="True" w190 {
              tunnel: w189 -> [w192 w195]
              tunnel: [w192 w194] -> w191
              tunnel: w188 -> [_ w193]
              frame False {
              }
              frame True {
                n48 = case shown="False" w193 {
                  tunnel: w195 -> [w197 w199]
                  tunnel: [w196 w199] -> w194
                  frame False {
                    n49 = Insert Into Array(array=w197, new element=action_typdef."Is BeamDump at Atmospheric Pressure?" ("action")) -> (w196:T2[])  [unwired: 1 in]
                  }
                  frame True {
                    # "Isolate HPBD"
                  }
                }
              }
            }
          }
          frame "OAP" {
            n50 = case shown="True" w200 {
              tunnel: w202 -> [w203 w205]
              tunnel: [w203 w204] -> w201
              frame False {
              }
              frame True {
                n51 = Insert Into Array(array=w205, new element=action_typdef."Is OAP at Atmospheric Pressure?" ("action")) -> (w204:T2[])  [unwired: 1 in]
              }
            }
          }
          frame "BTL" {
            n52 = case shown="True" w207 {
              tunnel: w209 -> [w210 w212]
              tunnel: [w210 w211] -> w208
              frame False {
              }
              frame True {
                n53 = Insert Into Array(array=w212, new element=action_typdef."Is BLT at Atmospheric Pressure" ("action")) -> (w211:T2[])  [unwired: 1 in]
              }
            }
          }
          frame "TARGET" {
            n54 = case shown="True" w214 {
              tunnel: w216 -> [w217 w219]
              tunnel: [w217 w218] -> w215
              frame False {
              }
              frame True {
                n55 = Insert Into Array(array=w219, new element=action_typdef."Is TARGET at Atmospheric Pressure?" ("action")) -> (w218:T2[])  [unwired: 1 in]
              }
            }
          }
          frame "BTL2" {
            n56 = case shown="True" w221 {
              tunnel: w223 -> [w224 w226]
              tunnel: [w224 w225] -> w222
              frame False {
              }
              frame True {
                n57 = Insert Into Array(array=w226, new element=action_typdef."Is BLT2 at Atmospheric Pressure?" ("action")) -> (w225:T2[])  [unwired: 1 in]
              }
            }
          }
          frame "HPD" {
            n58 = case shown="True" w230 {
              tunnel: w229 -> [w231 w233]
              tunnel: [w231 w232] -> w228
              frame False {
              }
              frame True {
                n59 = Insert Into Array(array=w233, new element=action_typdef."Is HPD at Atmospheric Pressure?" ("action")) -> (w232:T2[])  [unwired: 1 in]
              }
            }
          }
        }
      }
      frame "Check Chamber Pressures" {
        n60 = case shown="\"TARGET\"" w240 {
          tunnel: w239 -> [_ _ _ w254 _ _ _ _ _]
          tunnel: w238 -> [_ w243 w249 w256 w266 w273 w280 w287 w296]
          tunnel: w237 -> [_ w244 w248 w255 w268 w275 w282 w289 w295]
          tunnel: [w241 w242 w247 w257 w267 w274 w281 w288 w294] -> w236
          frame "False", Default {
            w241 = T2[] [enum."No Action"] items=["No Action", "Is EC GPM Mode ON?", "Is EC GPM Mode Off?", "Is EC GVM Mode ON?", "Is EC GVM Off?", "Is  EC GPM or GVM Mode ON?", "Is LB GPM Mode ON?", "Is LB GPM Mode Off?", "Is LB GVM Mode ON?", "Is LB GVM Mode Off?", "Is  LB GPM or GVM Mode ON?", "Is M123 Turbo Gate Valve Opened? ", "Is M123 Turbo Gate Valve Closed?", "Is OAP Turbo Gate Valve Opened?", "Is OAP Turbo Gate Valve Closed?", "Is BTLTurbo Gate Valve Opened?", "Is BTL Turbo Gate Valve Closed?", "Is TARGET Turbo Gate Valve 1Opened?", "Is TARGET1 Turbo Gate Valve Closed?", "Is TARGET Turbo Gate Valve 2 Opened?", "Is TAREGT2 Turbo Gate Valve Closed?", "Is BTL2 Turbo Gate Valve Opened?", "Is BTL2 Turbo Gate Valve Closed?", "Is HPD Turbo Gate Valve Opened?", "Is HPD Turbo Gate Valve Closed?", "Is COMP to M123 gate Valve Opened?", "Is COMP to M123 Valve Closed?", "Is HPBD Gate Valve Opened?", "Is HPBD Gate Valve Closed?", "Is M123 to OAP gate valve opened?", "Is M123 to OAP gate valve closed?", "Is OAP to BLT gate valve opened?", "Is OAP to BTL Gate Valve Closed?", "Is BLT to TARGET gate valve opened?", "Is BTL to TARGET Gate Valve Closed?", "Is TARGET to BLT2 gate valve opened?", "Is TARGET to BTL2 Gate Valve Closed?", "Is BLT2 to HPD gate valve opened?", "Is BTL2 to HPD Gate Valve Closed?", "Is COMP at Atmospheric Pressure?", "Is M123 at Atmospheric Pressure?", "Is BeamDump at Atmospheric Pressure?", "Is OAP at Atmospheric Pressure?", "Is BLT at Atmospheric Pressure", "Is TARGET at Atmospheric Pressure?", "Is BLT2 at Atmospheric Pressure?", "Is HPD at Atmospheric Pressure?", "Is the EC Roughing Pump ON?", "Is the EC Roughing Pump OFF?", "Does the EC Roughing Pump have a fault?", "Is the LB Roughing Pump ON?", "Is the LB Roughing Pump Off?", "Does the LB Roughing Pump have a fault?", "Is the EC Backing Pump ON?", "Is the EC Backing Pump OFF?", "Is the LB Backing Pump ON?", "Is the LB Backing Pump OFF?", "Does the EC Backing Pump have a fault?", "Does the LB Backing Pump have a fault?", "Is the EC Backing Pipe at Atmospheric Pressure", "Is the LB Backing Pipe at Atmospheric Pressure", "Is the EC Backing Manifold at Atmospheric Pressure", "s the LB Backing Manifold at Atmospheric Pressure?", "Is the EC Roughing Pipe at Atmospheric Pressure", "Is the LB Roughing Pipe at Atmospheric Pressure?", "Is the EC Roughing Manifold at Atmospheric Pressure", "Is the LB Roughing Manifold at Atmospheric Pressure", "Is LB Backing Manifold Valve Opened?", "Is EC Backing Manifold Valve Opened?", "Is LB Roughing Manifold Valve Opened?", "Is EC Roughing Manifold Valve Opened?", "Is COMP Roughing Valve Opened?", "Is M123 Roughing Valve Opened?", "Is M123 Roughing Valve Closed?", "Is OAP Roughing Valve Opened?", "Is OAP Roughing Valve Closed?", "Is HPBD Roughing Valve Opened?", "Is HPBD Roughing Valve Closed?", "Is BTL Roughing Valve Opened?", "Is BTL Roughing Valve Closed?", "Is TARGET Roughing Valve Opened?", "Is TARGET Roughing Valve Closed?", "Is BTL2 Roughing Valve Opened?", "Is BTL2 Roughing Valve Closed?", "Is HPD Roughing Valve Opened?", "Is HPD Roughing Valve Closed?", "Is COMP Turbo Backing Valve Opened?", "Is M123 Turbo Backing Valve Opened", "Is HPBD Turbo Backing Valve Opened?", "Is OAP Turbo Backing Valve Opened?", "Is BTL Turbo Backing Valve Opened?", "Is TARGET1 Turbo Backing Valve Opened?", "Is TARGET2 Turbo Backing Valve Opened?", "Is BTL2 Turbo Backing Valve Opened?", "Is HPD Turbo Backing Valve Opened?", "Is M123 Backing at MID-VAC?", "Is OAP Backing at MID-VAC?", "Is TARGET1 Backing at MID-VAC?", "Is TARGET2 Backing at MID-VAC?", "Is BTL Backing at MID-VAC?", "Is BTL2 Backing at MID-VAC?", "Is HPD Backing at MID-VAC?", "Is M123 Turbo in Normal Operation", "Is COMP Turbo in Normal Operation", "Is OAP Turbo in Normal Operation", "Is BTL Turbo in Normal Operation", "Is TARGET1 Turbo in Normal Operation", "Is TARGET2 Turbo in Normal Operation", "Is BTL2 Turbo in Normal Operation", "Is HPD Turbo in Normal Operation", "Is M123 at MID-VAC?", "Is OAP at MID-VAC?", "Is COMP at MID-VAC?", "Is BTL at MID-VAC?", "Is TARGET at MID-VAC?", "Is BTL2 at MID-VAC?", "Is HPD at MID-VAC?"]
          }
          frame "COMP" {
            n61 = case shown="True" w243 {
              tunnel: w244 -> [w245 w246]
              tunnel: [w245 w246] -> w242
              frame False {
              }
              frame True {
              }
            }
          }
          frame "M123" {
            n62 = case shown="True" w249 {
              tunnel: w248 -> [w250 w252]
              tunnel: [w250 w251] -> w247
              frame False {
              }
              frame True {
                n63 = Insert Into Array(array=w252, new element=action_typdef."Is M123 at MID-VAC?" ("action")) -> (w251:T2[])  [unwired: 1 in]
              }
            }
          }
          frame "HPBD" {
            n64 = case shown="True" w256 {
              tunnel: w255 -> [w258 w261]
              tunnel: [w258 w260] -> w257
              tunnel: w254 -> [_ w259]
              frame False {
              }
              frame True {
                n65 = case shown="False" w259 {
                  tunnel: w261 -> [w263 w265]
                  tunnel: [w262 w265] -> w260
                  frame False {
                    n66 = Insert Into Array(array=w263, new element=action_typdef."Is HPD at MID-VAC?" ("action")) -> (w262:T2[])  [unwired: 1 in]
                  }
                  frame True {
                    # "Isolate HPBD"
                  }
                }
              }
            }
          }
          frame "OAP" {
            n67 = case shown="True" w266 {
              tunnel: w268 -> [w269 w271]
              tunnel: [w269 w270] -> w267
              frame False {
              }
              frame True {
                n68 = Insert Into Array(array=w271, new element=action_typdef."Is OAP at MID-VAC?" ("action")) -> (w270:T2[])  [unwired: 1 in]
              }
            }
          }
          frame "BTL" {
            n69 = case shown="True" w273 {
              tunnel: w275 -> [w276 w278]
              tunnel: [w276 w277] -> w274
              frame False {
              }
              frame True {
                n70 = Insert Into Array(array=w278, new element=action_typdef."Is BTL at MID-VAC?" ("action")) -> (w277:T2[])  [unwired: 1 in]
              }
            }
          }
          frame "TARGET" {
            n71 = case shown="True" w280 {
              tunnel: w282 -> [w283 w285]
              tunnel: [w283 w284] -> w281
              frame False {
              }
              frame True {
                n72 = Insert Into Array(array=w285, new element=action_typdef."Is TARGET at MID-VAC?" ("action")) -> (w284:T2[])  [unwired: 1 in]
              }
            }
          }
          frame "BTL2" {
            n73 = case shown="True" w287 {
              tunnel: w289 -> [w290 w292]
              tunnel: [w290 w291] -> w288
              frame False {
              }
              frame True {
                n74 = Insert Into Array(array=w292, new element=action_typdef."Is BTL2 at MID-VAC?" ("action")) -> (w291:T2[])  [unwired: 1 in]
              }
            }
          }
          frame "HPD" {
            n75 = case shown="True" w296 {
              tunnel: w295 -> [w297 w299]
              tunnel: [w297 w298] -> w294
              frame False {
              }
              frame True {
                n76 = Insert Into Array(array=w299, new element=action_typdef."Is HPD Backing at MID-VAC?" ("action")) -> (w298:T2[])  [unwired: 1 in]
              }
            }
          }
        }
      }
      frame "Check Turbo Normal Operation" {
        n77 = case shown="\"TARGET\"" w306 {
          tunnel: w305 -> [_ _ _ w322 _ _ _ _ _]
          tunnel: w304 -> [_ w309 w317 w324 w332 w339 w346 w354 w363]
          tunnel: w303 -> [_ w310 w316 w323 w334 w341 w348 w356 w362]
          tunnel: [w307 w308 w315 w325 w333 w340 w347 w355 w361] -> w302
          frame "False", Default {
            w307 = T2[] [enum."No Action"] items=["No Action", "Is EC GPM Mode ON?", "Is EC GPM Mode Off?", "Is EC GVM Mode ON?", "Is EC GVM Off?", "Is  EC GPM or GVM Mode ON?", "Is LB GPM Mode ON?", "Is LB GPM Mode Off?", "Is LB GVM Mode ON?", "Is LB GVM Mode Off?", "Is  LB GPM or GVM Mode ON?", "Is M123 Turbo Gate Valve Opened? ", "Is M123 Turbo Gate Valve Closed?", "Is OAP Turbo Gate Valve Opened?", "Is OAP Turbo Gate Valve Closed?", "Is BTLTurbo Gate Valve Opened?", "Is BTL Turbo Gate Valve Closed?", "Is TARGET Turbo Gate Valve 1Opened?", "Is TARGET1 Turbo Gate Valve Closed?", "Is TARGET Turbo Gate Valve 2 Opened?", "Is TAREGT2 Turbo Gate Valve Closed?", "Is BTL2 Turbo Gate Valve Opened?", "Is BTL2 Turbo Gate Valve Closed?", "Is HPD Turbo Gate Valve Opened?", "Is HPD Turbo Gate Valve Closed?", "Is COMP to M123 gate Valve Opened?", "Is COMP to M123 Valve Closed?", "Is HPBD Gate Valve Opened?", "Is HPBD Gate Valve Closed?", "Is M123 to OAP gate valve opened?", "Is M123 to OAP gate valve closed?", "Is OAP to BLT gate valve opened?", "Is OAP to BTL Gate Valve Closed?", "Is BLT to TARGET gate valve opened?", "Is BTL to TARGET Gate Valve Closed?", "Is TARGET to BLT2 gate valve opened?", "Is TARGET to BTL2 Gate Valve Closed?", "Is BLT2 to HPD gate valve opened?", "Is BTL2 to HPD Gate Valve Closed?", "Is COMP at Atmospheric Pressure?", "Is M123 at Atmospheric Pressure?", "Is BeamDump at Atmospheric Pressure?", "Is OAP at Atmospheric Pressure?", "Is BLT at Atmospheric Pressure", "Is TARGET at Atmospheric Pressure?", "Is BLT2 at Atmospheric Pressure?", "Is HPD at Atmospheric Pressure?", "Is the EC Roughing Pump ON?", "Is the EC Roughing Pump OFF?", "Does the EC Roughing Pump have a fault?", "Is the LB Roughing Pump ON?", "Is the LB Roughing Pump Off?", "Does the LB Roughing Pump have a fault?", "Is the EC Backing Pump ON?", "Is the EC Backing Pump OFF?", "Is the LB Backing Pump ON?", "Is the LB Backing Pump OFF?", "Does the EC Backing Pump have a fault?", "Does the LB Backing Pump have a fault?", "Is the EC Backing Pipe at Atmospheric Pressure", "Is the LB Backing Pipe at Atmospheric Pressure", "Is the EC Backing Manifold at Atmospheric Pressure", "s the LB Backing Manifold at Atmospheric Pressure?", "Is the EC Roughing Pipe at Atmospheric Pressure", "Is the LB Roughing Pipe at Atmospheric Pressure?", "Is the EC Roughing Manifold at Atmospheric Pressure", "Is the LB Roughing Manifold at Atmospheric Pressure", "Is LB Backing Manifold Valve Opened?", "Is EC Backing Manifold Valve Opened?", "Is LB Roughing Manifold Valve Opened?", "Is EC Roughing Manifold Valve Opened?", "Is COMP Roughing Valve Opened?", "Is M123 Roughing Valve Opened?", "Is M123 Roughing Valve Closed?", "Is OAP Roughing Valve Opened?", "Is OAP Roughing Valve Closed?", "Is HPBD Roughing Valve Opened?", "Is HPBD Roughing Valve Closed?", "Is BTL Roughing Valve Opened?", "Is BTL Roughing Valve Closed?", "Is TARGET Roughing Valve Opened?", "Is TARGET Roughing Valve Closed?", "Is BTL2 Roughing Valve Opened?", "Is BTL2 Roughing Valve Closed?", "Is HPD Roughing Valve Opened?", "Is HPD Roughing Valve Closed?", "Is COMP Turbo Backing Valve Opened?", "Is M123 Turbo Backing Valve Opened", "Is HPBD Turbo Backing Valve Opened?", "Is OAP Turbo Backing Valve Opened?", "Is BTL Turbo Backing Valve Opened?", "Is TARGET1 Turbo Backing Valve Opened?", "Is TARGET2 Turbo Backing Valve Opened?", "Is BTL2 Turbo Backing Valve Opened?", "Is HPD Turbo Backing Valve Opened?", "Is M123 Backing at MID-VAC?", "Is OAP Backing at MID-VAC?", "Is TARGET1 Backing at MID-VAC?", "Is TARGET2 Backing at MID-VAC?", "Is BTL Backing at MID-VAC?", "Is BTL2 Backing at MID-VAC?", "Is HPD Backing at MID-VAC?", "Is M123 Turbo in Normal Operation", "Is COMP Turbo in Normal Operation", "Is OAP Turbo in Normal Operation", "Is BTL Turbo in Normal Operation", "Is TARGET1 Turbo in Normal Operation", "Is TARGET2 Turbo in Normal Operation", "Is BTL2 Turbo in Normal Operation", "Is HPD Turbo in Normal Operation", "Is M123 at MID-VAC?", "Is OAP at MID-VAC?", "Is COMP at MID-VAC?", "Is BTL at MID-VAC?", "Is TARGET at MID-VAC?", "Is BTL2 at MID-VAC?", "Is HPD at MID-VAC?"]
          }
          frame "COMP" {
            n78 = case shown="True" w309 {
              tunnel: w310 -> [w311 w314]
              tunnel: [w311 w312] -> w308
              frame False {
              }
              frame True {
                n79 = Insert Into Array(array=w314, new element=action_typdef."Is COMP Turbo in Normal Operation" ("action")) -> (w312:T2[])  [unwired: 1 in]
              }
            }
          }
          frame "M123" {
            n80 = case shown="True" w317 {
              tunnel: w316 -> [w318 w320]
              tunnel: [w318 w319] -> w315
              frame False {
              }
              frame True {
                n81 = Insert Into Array(array=w320, new element=action_typdef."Is M123 Turbo in Normal Operation" ("action")) -> (w319:T2[])  [unwired: 1 in]
              }
            }
          }
          frame "HPBD" {
            n82 = case shown="True" w324 {
              tunnel: w323 -> [w326 w329]
              tunnel: [w326 w328] -> w325
              tunnel: w322 -> [_ w327]
              frame False {
              }
              frame True {
                n83 = case shown="True" w327 {
                  tunnel: w329 -> [w330 w331]
                  tunnel: [w330 w331] -> w328
                  frame False {
                  }
                  frame True {
                    # "Isolate HPBD"
                  }
                }
              }
            }
          }
          frame "OAP" {
            n84 = case shown="True" w332 {
              tunnel: w334 -> [w335 w337]
              tunnel: [w335 w336] -> w333
              frame False {
              }
              frame True {
                n85 = Insert Into Array(array=w337, new element=action_typdef."Is OAP Turbo in Normal Operation" ("action")) -> (w336:T2[])  [unwired: 1 in]
              }
            }
          }
          frame "BTL" {
            n86 = case shown="True" w339 {
              tunnel: w341 -> [w342 w344]
              tunnel: [w342 w343] -> w340
              frame False {
              }
              frame True {
                n87 = Insert Into Array(array=w344, new element=action_typdef."Is BTL Turbo in Normal Operation" ("action")) -> (w343:T2[])  [unwired: 1 in]
              }
            }
          }
          frame "TARGET" {
            n88 = case shown="True" w346 {
              tunnel: w348 -> [w349 w352]
              tunnel: [w349 w351] -> w347
              frame False {
              }
              frame True {
                n89 = Insert Into Array(array=w352, new element #1=action_typdef."Is TARGET1 Turbo in Normal Operation" ("action"), new element #2=action_typdef."Is TARGET2 Turbo in Normal Operation" ("action")) -> (w351:T2[])  [unwired: 1 in]
              }
            }
          }
          frame "BTL2" {
            n90 = case shown="True" w354 {
              tunnel: w356 -> [w357 w359]
              tunnel: [w357 w358] -> w355
              frame False {
              }
              frame True {
                n91 = Insert Into Array(array=w359, new element=action_typdef."Is BTL2 Turbo in Normal Operation" ("action")) -> (w358:T2[])  [unwired: 1 in]
              }
            }
          }
          frame "HPD" {
            n92 = case shown="True" w363 {
              tunnel: w362 -> [w364 w366]
              tunnel: [w364 w365] -> w361
              frame False {
              }
              frame True {
                n93 = Insert Into Array(array=w366, new element=action_typdef."Is HPD Turbo in Normal Operation" ("action")) -> (w365:T2[])  [unwired: 1 in]
              }
            }
          }
        }
      }
      frame "Check Turbo Backing Valves" {
        n94 = case shown="\"HPD\"" w373 {
          tunnel: w372 -> [_ _ _ w389 _ _ _ _ _]
          tunnel: w371 -> [_ w376 w384 w391 w401 w408 w415 w423 w432]
          tunnel: w370 -> [_ w377 w383 w390 w403 w410 w417 w425 w431]
          tunnel: [w374 w375 w382 w392 w402 w409 w416 w424 w430] -> w369
          frame "False", Default {
            w374 = T2[] [enum."No Action"] items=["No Action", "Is EC GPM Mode ON?", "Is EC GPM Mode Off?", "Is EC GVM Mode ON?", "Is EC GVM Off?", "Is  EC GPM or GVM Mode ON?", "Is LB GPM Mode ON?", "Is LB GPM Mode Off?", "Is LB GVM Mode ON?", "Is LB GVM Mode Off?", "Is  LB GPM or GVM Mode ON?", "Is M123 Turbo Gate Valve Opened? ", "Is M123 Turbo Gate Valve Closed?", "Is OAP Turbo Gate Valve Opened?", "Is OAP Turbo Gate Valve Closed?", "Is BTLTurbo Gate Valve Opened?", "Is BTL Turbo Gate Valve Closed?", "Is TARGET Turbo Gate Valve 1Opened?", "Is TARGET1 Turbo Gate Valve Closed?", "Is TARGET Turbo Gate Valve 2 Opened?", "Is TAREGT2 Turbo Gate Valve Closed?", "Is BTL2 Turbo Gate Valve Opened?", "Is BTL2 Turbo Gate Valve Closed?", "Is HPD Turbo Gate Valve Opened?", "Is HPD Turbo Gate Valve Closed?", "Is COMP to M123 gate Valve Opened?", "Is COMP to M123 Valve Closed?", "Is HPBD Gate Valve Opened?", "Is HPBD Gate Valve Closed?", "Is M123 to OAP gate valve opened?", "Is M123 to OAP gate valve closed?", "Is OAP to BLT gate valve opened?", "Is OAP to BTL Gate Valve Closed?", "Is BLT to TARGET gate valve opened?", "Is BTL to TARGET Gate Valve Closed?", "Is TARGET to BLT2 gate valve opened?", "Is TARGET to BTL2 Gate Valve Closed?", "Is BLT2 to HPD gate valve opened?", "Is BTL2 to HPD Gate Valve Closed?", "Is COMP at Atmospheric Pressure?", "Is M123 at Atmospheric Pressure?", "Is BeamDump at Atmospheric Pressure?", "Is OAP at Atmospheric Pressure?", "Is BLT at Atmospheric Pressure", "Is TARGET at Atmospheric Pressure?", "Is BLT2 at Atmospheric Pressure?", "Is HPD at Atmospheric Pressure?", "Is the EC Roughing Pump ON?", "Is the EC Roughing Pump OFF?", "Does the EC Roughing Pump have a fault?", "Is the LB Roughing Pump ON?", "Is the LB Roughing Pump Off?", "Does the LB Roughing Pump have a fault?", "Is the EC Backing Pump ON?", "Is the EC Backing Pump OFF?", "Is the LB Backing Pump ON?", "Is the LB Backing Pump OFF?", "Does the EC Backing Pump have a fault?", "Does the LB Backing Pump have a fault?", "Is the EC Backing Pipe at Atmospheric Pressure", "Is the LB Backing Pipe at Atmospheric Pressure", "Is the EC Backing Manifold at Atmospheric Pressure", "s the LB Backing Manifold at Atmospheric Pressure?", "Is the EC Roughing Pipe at Atmospheric Pressure", "Is the LB Roughing Pipe at Atmospheric Pressure?", "Is the EC Roughing Manifold at Atmospheric Pressure", "Is the LB Roughing Manifold at Atmospheric Pressure", "Is LB Backing Manifold Valve Opened?", "Is EC Backing Manifold Valve Opened?", "Is LB Roughing Manifold Valve Opened?", "Is EC Roughing Manifold Valve Opened?", "Is COMP Roughing Valve Opened?", "Is M123 Roughing Valve Opened?", "Is M123 Roughing Valve Closed?", "Is OAP Roughing Valve Opened?", "Is OAP Roughing Valve Closed?", "Is HPBD Roughing Valve Opened?", "Is HPBD Roughing Valve Closed?", "Is BTL Roughing Valve Opened?", "Is BTL Roughing Valve Closed?", "Is TARGET Roughing Valve Opened?", "Is TARGET Roughing Valve Closed?", "Is BTL2 Roughing Valve Opened?", "Is BTL2 Roughing Valve Closed?", "Is HPD Roughing Valve Opened?", "Is HPD Roughing Valve Closed?", "Is COMP Turbo Backing Valve Opened?", "Is M123 Turbo Backing Valve Opened", "Is HPBD Turbo Backing Valve Opened?", "Is OAP Turbo Backing Valve Opened?", "Is BTL Turbo Backing Valve Opened?", "Is TARGET1 Turbo Backing Valve Opened?", "Is TARGET2 Turbo Backing Valve Opened?", "Is BTL2 Turbo Backing Valve Opened?", "Is HPD Turbo Backing Valve Opened?", "Is M123 Backing at MID-VAC?", "Is OAP Backing at MID-VAC?", "Is TARGET1 Backing at MID-VAC?", "Is TARGET2 Backing at MID-VAC?", "Is BTL Backing at MID-VAC?", "Is BTL2 Backing at MID-VAC?", "Is HPD Backing at MID-VAC?", "Is M123 Turbo in Normal Operation", "Is COMP Turbo in Normal Operation", "Is OAP Turbo in Normal Operation", "Is BTL Turbo in Normal Operation", "Is TARGET1 Turbo in Normal Operation", "Is TARGET2 Turbo in Normal Operation", "Is BTL2 Turbo in Normal Operation", "Is HPD Turbo in Normal Operation", "Is M123 at MID-VAC?", "Is OAP at MID-VAC?", "Is COMP at MID-VAC?", "Is BTL at MID-VAC?", "Is TARGET at MID-VAC?", "Is BTL2 at MID-VAC?", "Is HPD at MID-VAC?"]
          }
          frame "COMP" {
            n95 = case shown="True" w376 {
              tunnel: w377 -> [w378 w381]
              tunnel: [w378 w379] -> w375
              frame False {
              }
              frame True {
                n96 = Insert Into Array(array=w381, new element=action_typdef."Is COMP Turbo Backing Valve Opened?" ("action")) -> (w379:T2[])  [unwired: 1 in]
              }
            }
          }
          frame "M123" {
            n97 = case shown="True" w384 {
              tunnel: w383 -> [w385 w387]
              tunnel: [w385 w386] -> w382
              frame False {
              }
              frame True {
                n98 = Insert Into Array(array=w387, new element=action_typdef."Is M123 Turbo Backing Valve Opened" ("action")) -> (w386:T2[])  [unwired: 1 in]
              }
            }
          }
          frame "HPBD" {
            n99 = case shown="True" w391 {
              tunnel: w390 -> [w393 w396]
              tunnel: [w393 w395] -> w392
              tunnel: w389 -> [_ w394]
              frame False {
              }
              frame True {
                n100 = case shown="False" w394 {
                  tunnel: w396 -> [w398 w400]
                  tunnel: [w397 w400] -> w395
                  frame False {
                    n101 = Insert Into Array(array=w398, new element=action_typdef."Is HPBD Turbo Backing Valve Opened?" ("action")) -> (w397:T2[])  [unwired: 1 in]
                  }
                  frame True {
                    # "Isolate HPBD"
                  }
                }
              }
            }
          }
          frame "OAP" {
            n102 = case shown="True" w401 {
              tunnel: w403 -> [w404 w406]
              tunnel: [w404 w405] -> w402
              frame False {
              }
              frame True {
                n103 = Insert Into Array(array=w406, new element=action_typdef."Is OAP Turbo Backing Valve Opened?" ("action")) -> (w405:T2[])  [unwired: 1 in]
              }
            }
          }
          frame "BTL" {
            n104 = case shown="True" w408 {
              tunnel: w410 -> [w411 w413]
              tunnel: [w411 w412] -> w409
              frame False {
              }
              frame True {
                n105 = Insert Into Array(array=w413, new element=action_typdef."Is BTL Turbo Backing Valve Opened?" ("action")) -> (w412:T2[])  [unwired: 1 in]
              }
            }
          }
          frame "TARGET" {
            n106 = case shown="True" w415 {
              tunnel: w417 -> [w418 w421]
              tunnel: [w418 w420] -> w416
              frame False {
              }
              frame True {
                n107 = Insert Into Array(array=w421, new element #1=action_typdef."Is TARGET1 Turbo Backing Valve Opened?" ("action"), new element #2=action_typdef."Is TARGET2 Turbo Backing Valve Opened?" ("action")) -> (w420:T2[])  [unwired: 1 in]
              }
            }
          }
          frame "BTL2" {
            n108 = case shown="True" w423 {
              tunnel: w425 -> [w426 w428]
              tunnel: [w426 w427] -> w424
              frame False {
              }
              frame True {
                n109 = Insert Into Array(array=w428, new element=action_typdef."Is BTL2 Turbo Backing Valve Opened?" ("action")) -> (w427:T2[])  [unwired: 1 in]
              }
            }
          }
          frame "HPD" {
            n110 = case shown="True" w432 {
              tunnel: w431 -> [w433 w435]
              tunnel: [w433 w434] -> w430
              frame False {
              }
              frame True {
                n111 = Insert Into Array(array=w435, new element=action_typdef."Is HPD Turbo Backing Valve Opened?" ("action")) -> (w434:T2[])  [unwired: 1 in]
              }
            }
          }
        }
      }
      frame "Check MID-VAC on Chambers" {
        n112 = case shown="\"COMP\"" w442 {
          tunnel: w441 -> [_ _ _ w456 _ _ _ _ _]
          tunnel: w440 -> [_ w445 w451 w458 w466 w473 w480 w488 w497]
          tunnel: w439 -> [_ w446 w450 w457 w468 w475 w482 w490 w496]
          tunnel: [w443 w444 w449 w459 w467 w474 w481 w489 w495] -> w438
          frame "False", Default {
            w443 = T2[] [enum."No Action"] items=["No Action", "Is EC GPM Mode ON?", "Is EC GPM Mode Off?", "Is EC GVM Mode ON?", "Is EC GVM Off?", "Is  EC GPM or GVM Mode ON?", "Is LB GPM Mode ON?", "Is LB GPM Mode Off?", "Is LB GVM Mode ON?", "Is LB GVM Mode Off?", "Is  LB GPM or GVM Mode ON?", "Is M123 Turbo Gate Valve Opened? ", "Is M123 Turbo Gate Valve Closed?", "Is OAP Turbo Gate Valve Opened?", "Is OAP Turbo Gate Valve Closed?", "Is BTLTurbo Gate Valve Opened?", "Is BTL Turbo Gate Valve Closed?", "Is TARGET Turbo Gate Valve 1Opened?", "Is TARGET1 Turbo Gate Valve Closed?", "Is TARGET Turbo Gate Valve 2 Opened?", "Is TAREGT2 Turbo Gate Valve Closed?", "Is BTL2 Turbo Gate Valve Opened?", "Is BTL2 Turbo Gate Valve Closed?", "Is HPD Turbo Gate Valve Opened?", "Is HPD Turbo Gate Valve Closed?", "Is COMP to M123 gate Valve Opened?", "Is COMP to M123 Valve Closed?", "Is HPBD Gate Valve Opened?", "Is HPBD Gate Valve Closed?", "Is M123 to OAP gate valve opened?", "Is M123 to OAP gate valve closed?", "Is OAP to BLT gate valve opened?", "Is OAP to BTL Gate Valve Closed?", "Is BLT to TARGET gate valve opened?", "Is BTL to TARGET Gate Valve Closed?", "Is TARGET to BLT2 gate valve opened?", "Is TARGET to BTL2 Gate Valve Closed?", "Is BLT2 to HPD gate valve opened?", "Is BTL2 to HPD Gate Valve Closed?", "Is COMP at Atmospheric Pressure?", "Is M123 at Atmospheric Pressure?", "Is BeamDump at Atmospheric Pressure?", "Is OAP at Atmospheric Pressure?", "Is BLT at Atmospheric Pressure", "Is TARGET at Atmospheric Pressure?", "Is BLT2 at Atmospheric Pressure?", "Is HPD at Atmospheric Pressure?", "Is the EC Roughing Pump ON?", "Is the EC Roughing Pump OFF?", "Does the EC Roughing Pump have a fault?", "Is the LB Roughing Pump ON?", "Is the LB Roughing Pump Off?", "Does the LB Roughing Pump have a fault?", "Is the EC Backing Pump ON?", "Is the EC Backing Pump OFF?", "Is the LB Backing Pump ON?", "Is the LB Backing Pump OFF?", "Does the EC Backing Pump have a fault?", "Does the LB Backing Pump have a fault?", "Is the EC Backing Pipe at Atmospheric Pressure", "Is the LB Backing Pipe at Atmospheric Pressure", "Is the EC Backing Manifold at Atmospheric Pressure", "s the LB Backing Manifold at Atmospheric Pressure?", "Is the EC Roughing Pipe at Atmospheric Pressure", "Is the LB Roughing Pipe at Atmospheric Pressure?", "Is the EC Roughing Manifold at Atmospheric Pressure", "Is the LB Roughing Manifold at Atmospheric Pressure", "Is LB Backing Manifold Valve Opened?", "Is EC Backing Manifold Valve Opened?", "Is LB Roughing Manifold Valve Opened?", "Is EC Roughing Manifold Valve Opened?", "Is COMP Roughing Valve Opened?", "Is M123 Roughing Valve Opened?", "Is M123 Roughing Valve Closed?", "Is OAP Roughing Valve Opened?", "Is OAP Roughing Valve Closed?", "Is HPBD Roughing Valve Opened?", "Is HPBD Roughing Valve Closed?", "Is BTL Roughing Valve Opened?", "Is BTL Roughing Valve Closed?", "Is TARGET Roughing Valve Opened?", "Is TARGET Roughing Valve Closed?", "Is BTL2 Roughing Valve Opened?", "Is BTL2 Roughing Valve Closed?", "Is HPD Roughing Valve Opened?", "Is HPD Roughing Valve Closed?", "Is COMP Turbo Backing Valve Opened?", "Is M123 Turbo Backing Valve Opened", "Is HPBD Turbo Backing Valve Opened?", "Is OAP Turbo Backing Valve Opened?", "Is BTL Turbo Backing Valve Opened?", "Is TARGET1 Turbo Backing Valve Opened?", "Is TARGET2 Turbo Backing Valve Opened?", "Is BTL2 Turbo Backing Valve Opened?", "Is HPD Turbo Backing Valve Opened?", "Is M123 Backing at MID-VAC?", "Is OAP Backing at MID-VAC?", "Is TARGET1 Backing at MID-VAC?", "Is TARGET2 Backing at MID-VAC?", "Is BTL Backing at MID-VAC?", "Is BTL2 Backing at MID-VAC?", "Is HPD Backing at MID-VAC?", "Is M123 Turbo in Normal Operation", "Is COMP Turbo in Normal Operation", "Is OAP Turbo in Normal Operation", "Is BTL Turbo in Normal Operation", "Is TARGET1 Turbo in Normal Operation", "Is TARGET2 Turbo in Normal Operation", "Is BTL2 Turbo in Normal Operation", "Is HPD Turbo in Normal Operation", "Is M123 at MID-VAC?", "Is OAP at MID-VAC?", "Is COMP at MID-VAC?", "Is BTL at MID-VAC?", "Is TARGET at MID-VAC?", "Is BTL2 at MID-VAC?", "Is HPD at MID-VAC?"]
          }
          frame "COMP" {
            n113 = case shown="True" w445 {
              tunnel: w446 -> [w447 w448]
              tunnel: [w447 w448] -> w444
              frame False {
              }
              frame True {
              }
            }
          }
          frame "M123" {
            n114 = case shown="True" w451 {
              tunnel: w450 -> [w452 w454]
              tunnel: [w452 w453] -> w449
              frame False {
              }
              frame True {
                n115 = Insert Into Array(array=w454, new element=action_typdef."Is M123 Backing at MID-VAC?" ("action")) -> (w453:T2[])  [unwired: 1 in]
              }
            }
          }
          frame "HPBD" {
            n116 = case shown="False" w458 {
              tunnel: w457 -> [w460 w463]
              tunnel: [w460 w462] -> w459
              tunnel: w456 -> [_ w461]
              frame False {
              }
              frame True {
                n117 = case shown="False" w461 {
                  tunnel: w463 -> [w464 w465]
                  tunnel: [w464 w465] -> w462
                  frame False {
                  }
                  frame True {
                    # "Isolate HPBD"
                  }
                }
              }
            }
          }
          frame "OAP" {
            n118 = case shown="True" w466 {
              tunnel: w468 -> [w469 w471]
              tunnel: [w469 w470] -> w467
              frame False {
              }
              frame True {
                n119 = Insert Into Array(array=w471, new element=action_typdef."Is OAP Backing at MID-VAC?" ("action")) -> (w470:T2[])  [unwired: 1 in]
              }
            }
          }
          frame "BTL" {
            n120 = case shown="True" w473 {
              tunnel: w475 -> [w476 w478]
              tunnel: [w476 w477] -> w474
              frame False {
              }
              frame True {
                n121 = Insert Into Array(array=w478, new element=action_typdef."Is BTL Backing at MID-VAC?" ("action")) -> (w477:T2[])  [unwired: 1 in]
              }
            }
          }
          frame "TARGET" {
            n122 = case shown="True" w480 {
              tunnel: w482 -> [w483 w486]
              tunnel: [w483 w485] -> w481
              frame False {
              }
              frame True {
                n123 = Insert Into Array(array=w486, new element #1=action_typdef."Is TARGET1 Backing at MID-VAC?" ("action"), new element #2=action_typdef."Is TARGET2 Backing at MID-VAC?" ("action")) -> (w485:T2[])  [unwired: 1 in]
              }
            }
          }
          frame "BTL2" {
            n124 = case shown="True" w488 {
              tunnel: w490 -> [w491 w493]
              tunnel: [w491 w492] -> w489
              frame False {
              }
              frame True {
                n125 = Insert Into Array(array=w493, new element=action_typdef."Is BTL2 Backing at MID-VAC?" ("action")) -> (w492:T2[])  [unwired: 1 in]
              }
            }
          }
          frame "HPD" {
            n126 = case shown="True" w497 {
              tunnel: w496 -> [w498 w500]
              tunnel: [w498 w499] -> w495
              frame False {
              }
              frame True {
                n127 = Insert Into Array(array=w500, new element=action_typdef."Is HPD Backing at MID-VAC?" ("action")) -> (w499:T2[])  [unwired: 1 in]
              }
            }
          }
        }
      }
    }
  }
  n128 = Empty Array?(array=w6) -> (empty?=w9:bool)
  n129 = Empty Array?(array=w3) -> (empty?=w4:bool)
  n130 = Select(t=w7, s=w9, f=w6) -> (s? t:f=→"Action Array Out":T2[])
  n131 = Select(t=w2, s=w4, f=w3) -> (s? t:f=→"Command Array Out":T1[])
